vi "Get Kinematic Parameters.vi"(11 "NI_Robotics_Link in":refnum<class "NI_Robotics_Link.lvclass">) -> (0 "Rotation Angle":dbl, 1 "Offset Distance":dbl, 2 "Length":dbl, 3 "Twist Angle":dbl, 4 "Joint Coordinate Offset":dbl)   [LabVIEW 2017, in "NI_Robotics_Link.lvclass"]
uses:
  <vilib>/robotics/Kinematics/Link/NI_Robotics_Link.lvclass
  <vilib>/robotics/Kinematics/Link/NI_Robotics_Link.lvclass/NI_Robotics_Link.ctl
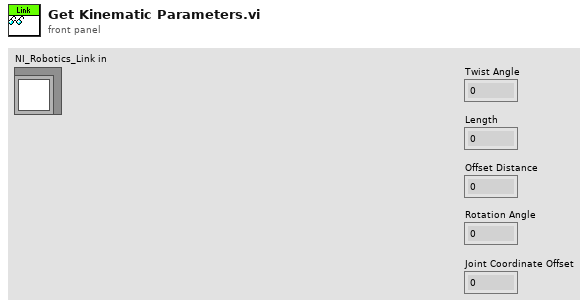
[diagram p1: front panel]
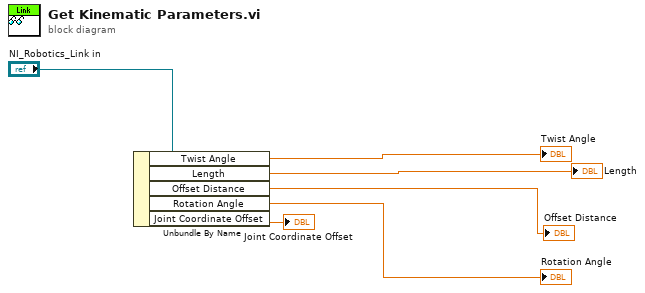
[diagram p0: block diagram]
diagram:
  n1 = Unbundle By Name("NI_Robotics_Link in") -> ("Twist Angle"=→"Twist Angle":dbl, "Length"=→"Length":dbl, "Offset Distance"=→"Offset Distance":dbl, "Rotation Angle"=→"Rotation Angle":dbl, "Joint Coordinate Offset"=→"Joint Coordinate Offset":dbl)
